vi "FTW-Regex-Execute.vi"(0 "Regex":refnum<class "FTW-Regex.lvclass">, 5 "Subject String":string, 7 "Starting Offset":i32, 9 "Submatch Buffer Size":i32=100, 11 "error in":errorcluster) -> (4 "Regex out":refnum<class "FTW-Regex.lvclass">, 6 "Whole Match Begin":i32, 8 "Offset after Match":i32, 10 "Submatches":i32[](array[numeric]), 14 "Callouts":T1(array[cluster]), 15 "error out":errorcluster)   [LabVIEW 2014, in "FTW-Regex.lvclass"]
uses:
  FTW-Regex.lvclass
  FTW-Regex.lvclass/FTW-Regex.ctl
  error/FTW-ERR-ThrowError.vi
  error/FTW-ERR-NoErrorConstant.vi
  error/FTW-ERR-CallChain.vi
  string/FTW-STR-ReplaceWhitespace.vi
panel:
  # "Inputs"
  # "Outputs"
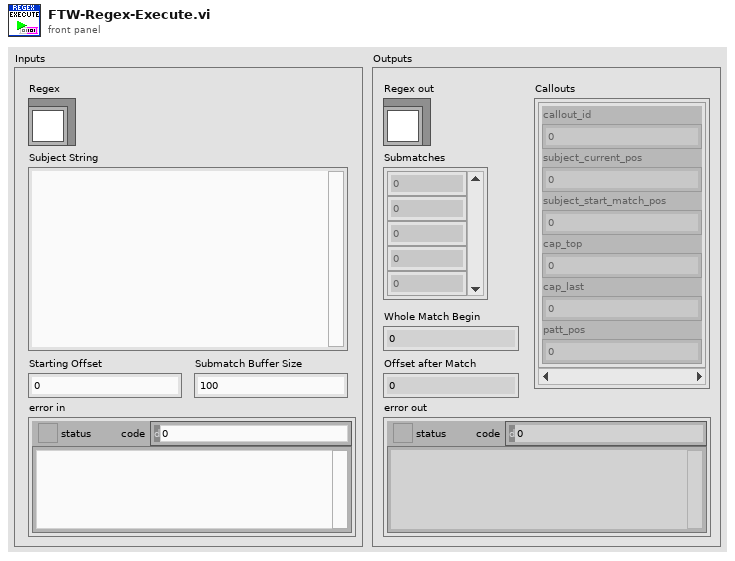
[diagram p1: front panel]
types:
  T1 = cluster{"callout_id":i32, "subject_current_pos":i32, "subject_start_match_pos":i32, "cap_top":i32, "cap_last":i32, "patt_pos":i32}[]
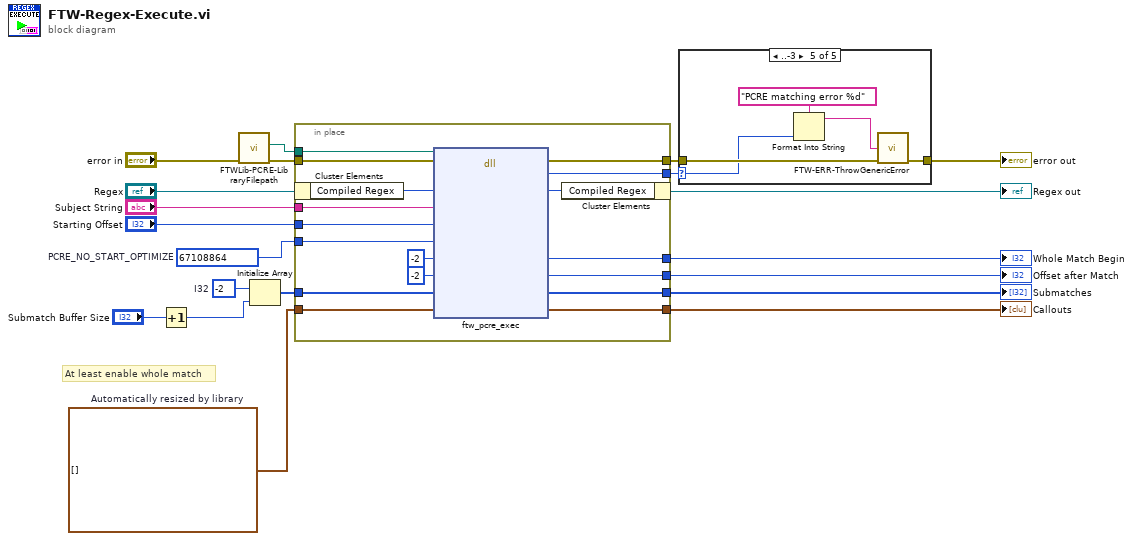
[diagram p0: block diagram]
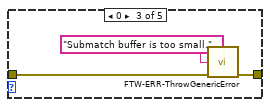
[diagram p4: hidden frame]
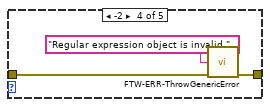
[diagram p5: hidden frame]
diagram:
  w4 = -2  # I32
  w11 = T1 []  # Automatically resized by library
  w12 = 67108864  # PCRE_NO_START_OPTIMIZE
  # "At least enable whole match"
  n1 = Increment(x="Submatch Buffer Size") -> (x+1=w1:i32)
  n2 = call "FTWLib-PCRE-LibraryFilepath.vi"("error in"="error in") -> ("error out"=w18:errorcluster, "PCRE Library Filepath"=w19:path)  [unwired: 8 in, 1 out]
  n3 = Initialize Array(w4, w1) -> (w3:i32[])
  n4 = in-place {
    in-place-border: [w37] -> w6
    in-place-border: w19 -> [w36]
    in-place-border: w18 -> [w35]
    in-place-border: "Subject String" -> [w32]
    in-place-border: "Starting Offset" -> [w31]
    in-place-border: [w25] -> w13
    in-place-border: w12 -> [w30]
    in-place-border: w3 -> [w27]
    in-place-border: w11 -> [w26]
    in-place-border: [w24] -> w10
    in-place-border: [w23] -> w9
    in-place-border: [w22] -> w8
    in-place-border: [w21] -> w5
    n5 = in-place-cluster #1("Regex") -> ("Compiled Regex"=w34:u64)
    n6 = dll-call lib="?" fn="ftw_pcre_exec"(path in=w36, error in=w35, "Compiled Regex"=w34, "Subject String"=w32, "Starting Offset"=w31, "Options"=w30, "Match Begin"=-2, "Match End"=-2, "Submatch Buffer"=w27, "Callout Buffer"=w26) -> (error out=w37:errorcluster, "Return Value"=w22:i64, "Compiled Regex"=w33:u64, "Match Begin"=w21:i32, "Match End"=w25:i32, "Submatch Buffer"=w24:i32[], "Callout Buffer"=w23:T1)  [unwired: 4 in, 1 out]
    n7 = in-place-cluster #1("Compiled Regex"=w33) -> (→"Regex out":refnum<class "FTW-Regex.lvclass">)
  }
  "Offset after Match" <- w13
  "Submatches" <- w10
  "Callouts" <- w9
  "Whole Match Begin" <- w5
  n8 = case shown="..-3" w8 {
    selector: w8 -> [_ _ _ _ w48]
    tunnel: [w38 w39 w41 w44 w49] -> w7
    tunnel: w6 -> [w38 w39 w42 w45 w50]
    frame 1.. {
      # "Match found and no error."
    }
    frame -1 {
      # "PCRE_ERROR_NOMATCH\nDon't treat this as an error!"
    }
    frame 0 {
      n9 = call "FTW-ERR-ThrowGenericError.vi"("Error Message"="Submatch buffer is too small.", "error in"=w42) -> ("error out"=w41:errorcluster)  [unwired: 13 in]
    }
    frame -2 {
      n10 = call "FTW-ERR-ThrowGenericError.vi"("Error Message"="Regular expression object is invalid.", "error in"=w45) -> ("error out"=w44:errorcluster)  [unwired: 13 in]
    }
    frame ..-3 {
      n11 = Format Into String(format string="PCRE matching error %d" ("Error Message"), w48) -> (resulting string=w47:string)  [unwired: 2 in, 1 out]
      n12 = call "FTW-ERR-ThrowGenericError.vi"("Error Message"=w47, "error in"=w50) -> ("error out"=w49:errorcluster)  [unwired: 13 in]
    }
  }
  "error out" <- w7
